vi "ConfigOutputEnableV01.vi"(8 "error in (no error)":errorcluster, 11 "ClassIn":refnum<class "Keysight335XX.lvclass">) -> (0 "error out":errorcluster, 3 "ClassOut":refnum<class "Keysight335XX.lvclass">)   [LabVIEW 2014, in "FGenPlugins.lvlib" / "Keysight335XX.lvclass"]
uses:
  Keysight335XX.lvclass
  <instrlib>/Agilent 3352X Series/Agilent 3352X Series.lvlib
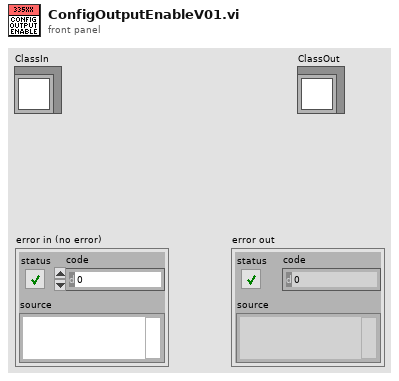
[diagram p1: front panel]
types:
  T1 = typedef "FGenPlugins.lvlib/NISTFGenPluginsBase.lvclass/ChannelParamElement.ctl" = cluster{"sName":string, "eOperateMode":u16, "bEnabled":bool, "eOutputMode":u16, "iIndex":i32, "iNameBufferSize":i32, "fGain":dbl}
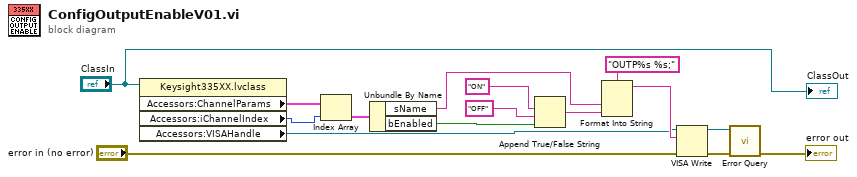
[diagram p0: block diagram]
diagram:
  n1 = property class="Keysight335XX.lvclass"(reference="ClassIn") -> ("Accessors:ChannelParams"=w7:T1[], "Accessors:iChannelIndex"=w5:i32, "Accessors:VISAHandle"=w2:refnum<visa-resource-name>)  [unwired: 1 in, 2 out]
  n2 = Index Array(array=w7, index=w5) -> (element=w6:T1)
  n3 = Unbundle By Name(w6) -> ("sName"=w3:string, "bEnabled"=w4:bool)
  n4 = Append True/False String(1:w4, 2:"OFF", 3:"ON") -> (0:w10:string)  [unwired: 1 out]
  n5 = Format Into String(format string="OUTP%s %s;", w3, w10) -> (resulting string=w12:string)  [unwired: 2 in, 1 out]
  n6 = VISA Write(VISA resource name=w2, write buffer=w12, error in (no error)="error in (no error)") -> (VISA resource name out=w13:refnum<visa-resource-name>, error out=w14:errorcluster)  [unwired: 1 out]
  n7 = call <instrlib>:"Error Query.vi"("error in (no error)"=w14, "VISA resource name"=w13) -> ("error out"=→"error out":errorcluster)  [unwired: 9 out]
  "ClassOut" <- "ClassIn"
